vi "MCU.vi"(11 "Shared_strings":string[][](array[string])) -> ()   [LabVIEW 2018]
uses:
  Global Variables.vi
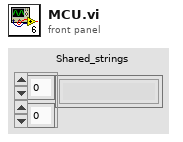
[diagram p1: front panel]
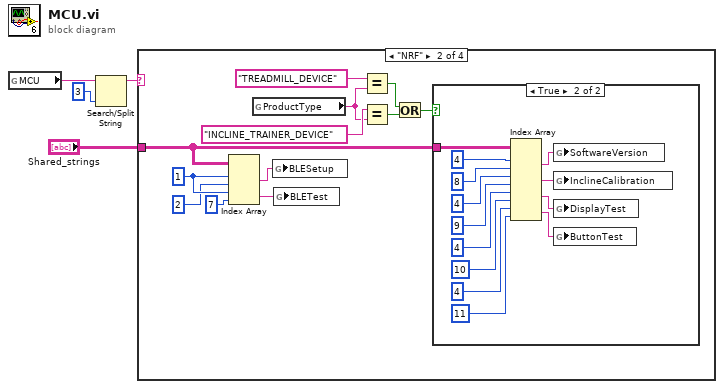
[diagram p0: block diagram]
diagram:
  n1 = global read "Global Variables.vi" "MCU"() -> (w3:string)
  n2 = Search/Split String(string=w3, offset (0)=3) -> (substring before match=w1:string)  [unwired: 1 in, 2 out]
  n3 = case shown="\"NRF\"" w1 {
    tunnel: "Shared_strings" -> [_ w11 _ _]
    frame "PSO", Default {
    }
    frame "NRF" {
      w16 = 1
      n4 = Index Array(array=w11, index (row) #1=w16, index (col) #1=2, index (row) #2=w16, index (col) #2=7) -> (element #1=w13:string, element #2=w12:string)
      n5 = global read "Global Variables.vi" "ProductType"() -> (w8:string)
      n6 = global write "Global Variables.vi" "BLESetup"(w13) -> ()
      n7 = global write "Global Variables.vi" "BLETest"(w12) -> ()
      n8 = Equal?(x="TREADMILL_DEVICE" ("y"), y=w8) -> (x = y?=w7:bool)
      n9 = Equal?(x="INCLINE_TRAINER_DEVICE" ("y"), y=w8) -> (x = y?=w6:bool)
      n10 = Or(x=w7, y=w6) -> (x .or. y?=w5:bool)
      n11 = case shown="True" w5 {
        tunnel: w11 -> [_ w29]
        frame False {
        }
        frame True {
          n12 = Index Array(array=w29, index (row) #1=4, index (col) #1=8, index (row) #2=4, index (col) #2=9, index (row) #3=4, index (col) #3=10, index (row) #4=4, index (col) #4=11) -> (element #1=w28:string, element #2=w27:string, element #3=w26:string, element #4=w25:string)
          n13 = global write "Global Variables.vi" "SoftwareVersion"(w28) -> ()
          n14 = global write "Global Variables.vi" "InclineCalibration"(w27) -> ()
          n15 = global write "Global Variables.vi" "DisplayTest"(w26) -> ()
          n16 = global write "Global Variables.vi" "ButtonTest"(w25) -> ()
        }
      }
    }
    frame "REN" {
    }
    frame "ZIL" {
    }
  }
